vi "get_numeric_value.vi"(3 "error in (no error)":errorcluster, 4 "field name":string, 5 "metadata JSON string":string) -> (0 "error out":errorcluster, 2 "field value":dbl format="%#_13g")   [LabVIEW 2013, in "Rinocloud Library.lvlib"]
uses:
  i3 JSON/JSON Parsing/Get Object Parameter Files/Get Object Parameter - Numeric.vi
  Rinocloud Library.lvlib
  i3 JSON/i3-json.lvlib
panel:
  out "found":bool
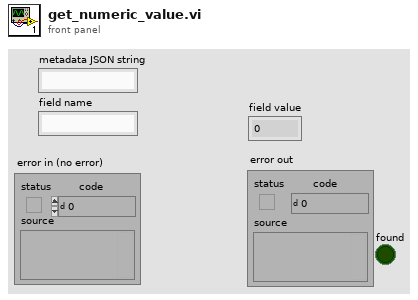
[diagram p1: front panel]
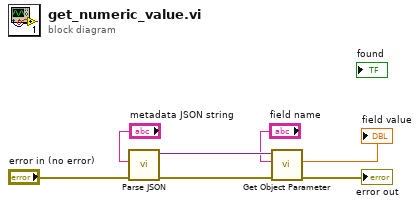
[diagram p0: block diagram]
diagram:
  n1 = call "Parse JSON.vi"("error in (no error)"="error in (no error)", "JSON String"="metadata JSON string") -> ("error out"=w5:errorcluster, "JSON Tree"=w6:variant)  [unwired: 6 in, 2 out]
  n2 = call-poly "Get Object Parameter.vi"("error in (no error)"=w5, "Parameter Name"="field name", "JSON Tree In (JSON Object)"=w6) -> ("error out"=→"error out":errorcluster, "Double Value"=→"field value":dbl)  [unwired: 5 in, 2 out]
